vi "Toggle.vi"(10 "InitialState":bool, 11 "FlashInput":bool) -> (3 "Toggled":bool)   [LabVIEW 2020]
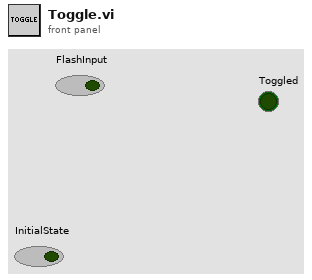
[diagram p1: front panel]
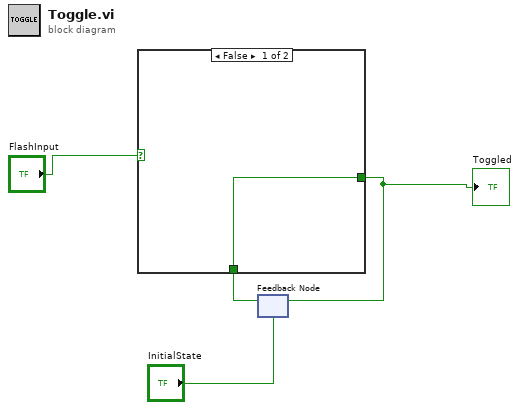
[diagram p0: block diagram]
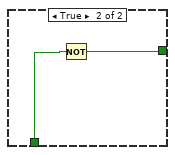
[diagram p2: hidden frame]
diagram:
  n1 = feedback #1("InitialState") -> (w2:bool)
  n2 = case shown="False" "FlashInput" {
    tunnel: [w5 w7] -> w3
    tunnel: w2 -> [w5 w6]
    frame False {
    }
    frame True {
      n3 = Not(x=w6) -> (.not. x?=w7:bool)
    }
  }
  "Toggled" <- w3
  n4 = feedback-in #1(w3) -> ()
